vi "Initialize.vi"(7 "Process ID":string, 8 "error in (no error)":errorcluster, 10 "Device Item Ref":T1=18446744073709551615 format="%.0x", 11 "Output Process in":refnum<class "Sine Process.lvclass">) -> (0 "error out":errorcluster, 3 "Output Process out":refnum<class "Sine Process.lvclass">)   [LabVIEW 2019, in "TimingDRV Engine.lvlib" / "Sine Process.lvclass"]
uses:
  Sine Process.lvclass
  <vilib>/NI VeriStand/Custom Device API/Custom Device Item Ref.ctl
  Parent Classes/Process/Process.lvclass
  <vilib>/NI VeriStand/Custom Device API/Custom Device API.lvlib
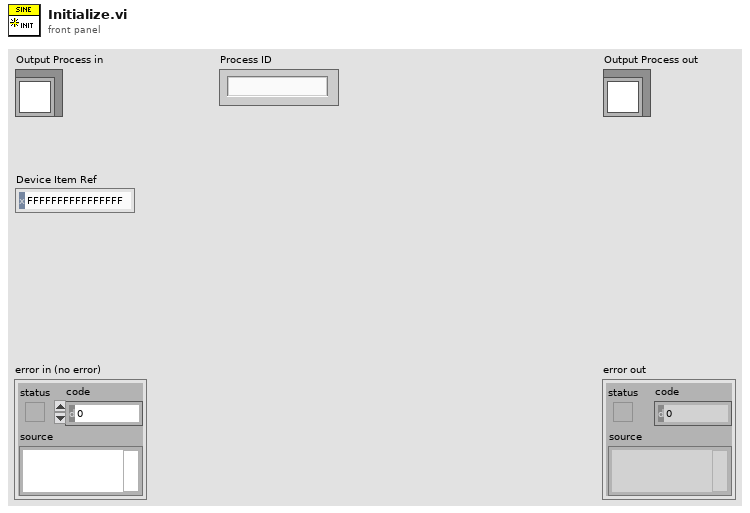
[diagram p1: front panel]
types:
  T1 = typedef "Custom Device API.lvlib/Custom Device Item Ref.ctl" = u64
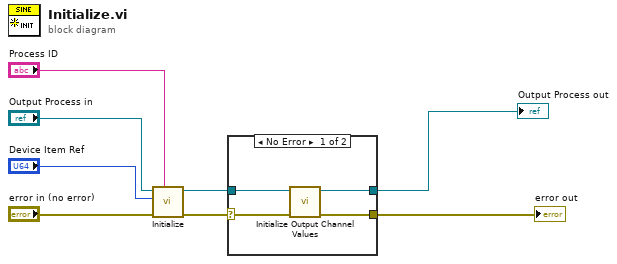
[diagram p0: block diagram]
diagram:
  n1 = call-parent "Initialize.vi"("Process ID"="Process ID", "error in (no error)"="error in (no error)", "Device Item Ref"="Device Item Ref", "Process in"="Output Process in") -> ("error out"=w4:errorcluster, "Process out"=w3:refnum<class "Sine Process.lvclass">)  [unwired: 6 in]
  n2 = case shown="No Error" w4 {
    selector: w4 -> [w11 w13]
    tunnel: w3 -> [w12 w14]
    tunnel: [w10 w13] -> w2
    tunnel: [w9 w14] -> w1
    frame No Error {
      n3 = call "Initialize Output Channel Values.vi"("error in (no error)"=w11, "Output Process in"=w12) -> ("error out"=w10:errorcluster, "Output Process out"=w9:refnum<class "Sine Process.lvclass">)  [unwired: 8 in]
    }
    frame Error {
    }
  }
  "error out" <- w2
  "Output Process out" <- w1
